vi "Core Actor - Init User Events.vi"(8 "error in (no error)":errorcluster, 11 "Interface_Class in":refnum<class "Abstraction_Interface_Class.lvclass">) -> (0 "error out":errorcluster, 3 "Interface_Class out":refnum<class "Abstraction_Interface_Class.lvclass">)   [LabVIEW 2023, in "Abstraction_Interface.lvlib" / "Abstraction_Interface_Class.lvclass"]
uses:
  Abstraction_Interface_Class.lvclass
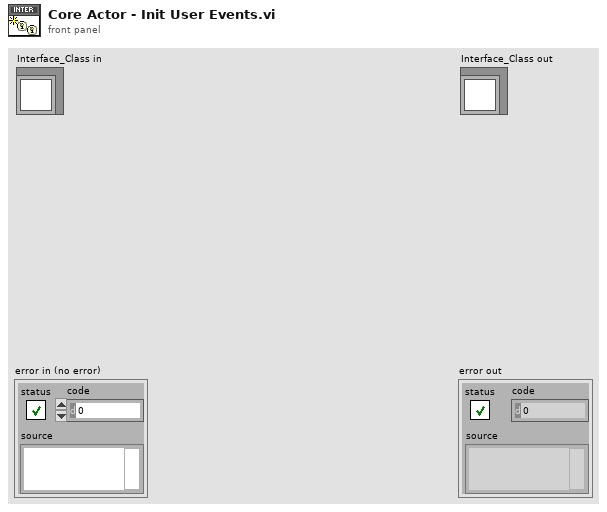
[diagram p1: front panel]
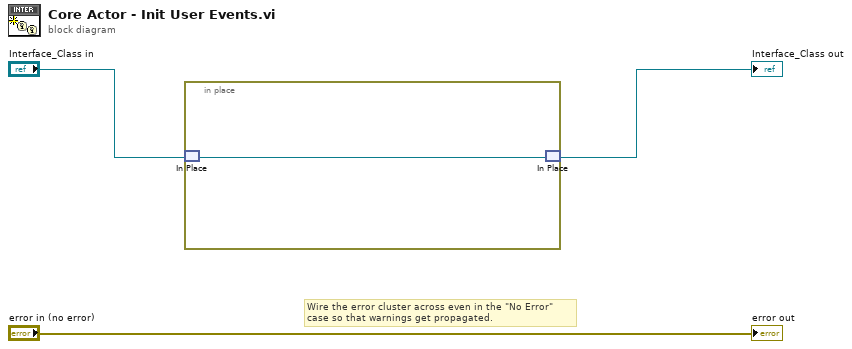
[diagram p0: block diagram]
diagram:
  # "Wire the error cluster across even in the \"No Error\"\ncase so that warnings get propagated."
  n1 = in-place {
    n2 = in-place-match #1("Interface_Class in") -> (w4:refnum<class "Abstraction_Interface_Class.lvclass">)
    n3 = in-place-match #1(w4) -> (→"Interface_Class out":refnum<class "Abstraction_Interface_Class.lvclass">)
  }
  "error out" <- "error in (no error)"
